vi "Circular Buffer(2D Wfm).vi"(7 "Buffer Size":T3, 8 "error in (no error)":errorcluster, 9 "Read Size":i32, 10 "Operation":T1, 11 "Data In":waveform(dbl)[](array[waveform])) -> (0 "error out":errorcluster, 1 "Elements Remaining":i32, 2 "Buffer Status":T2, 3 "Data Out":waveform(dbl)[](array[waveform]))   [LabVIEW 2016, in "Circular Buffer.lvlib"]
doc: "This VI implements a circular buffer which data can be written to and read from. There can only be one buffer per data type at once, but you can have multiple buffers of different types at the same time. For example, you can have a buffer of Wfm data types as well as I32s in the same VI. You cannot have two independent buffers of I32s."
uses:
  Circular Buffer.lvlib
  Controls/Circular Buffer Status.ctl
  Controls/Circular Buffer Operations.ctl
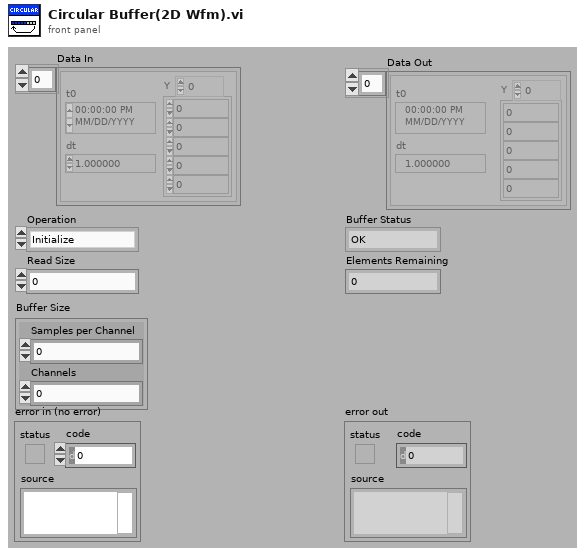
[diagram p1: front panel]
types:
  T1 = typedef "Circular Buffer.lvlib/Circular Buffer Operations.ctl" = enum16{"Initialize", "Get Backlog", "Write", "Read (continuous)", "Read (most recent)"}
  T2 = typedef "Circular Buffer.lvlib/Circular Buffer Status.ctl" = enum16{"OK", "Overflow", "Underflow"}
  T3 = cluster{"Samples per Channel":u32, "Channels":u32}
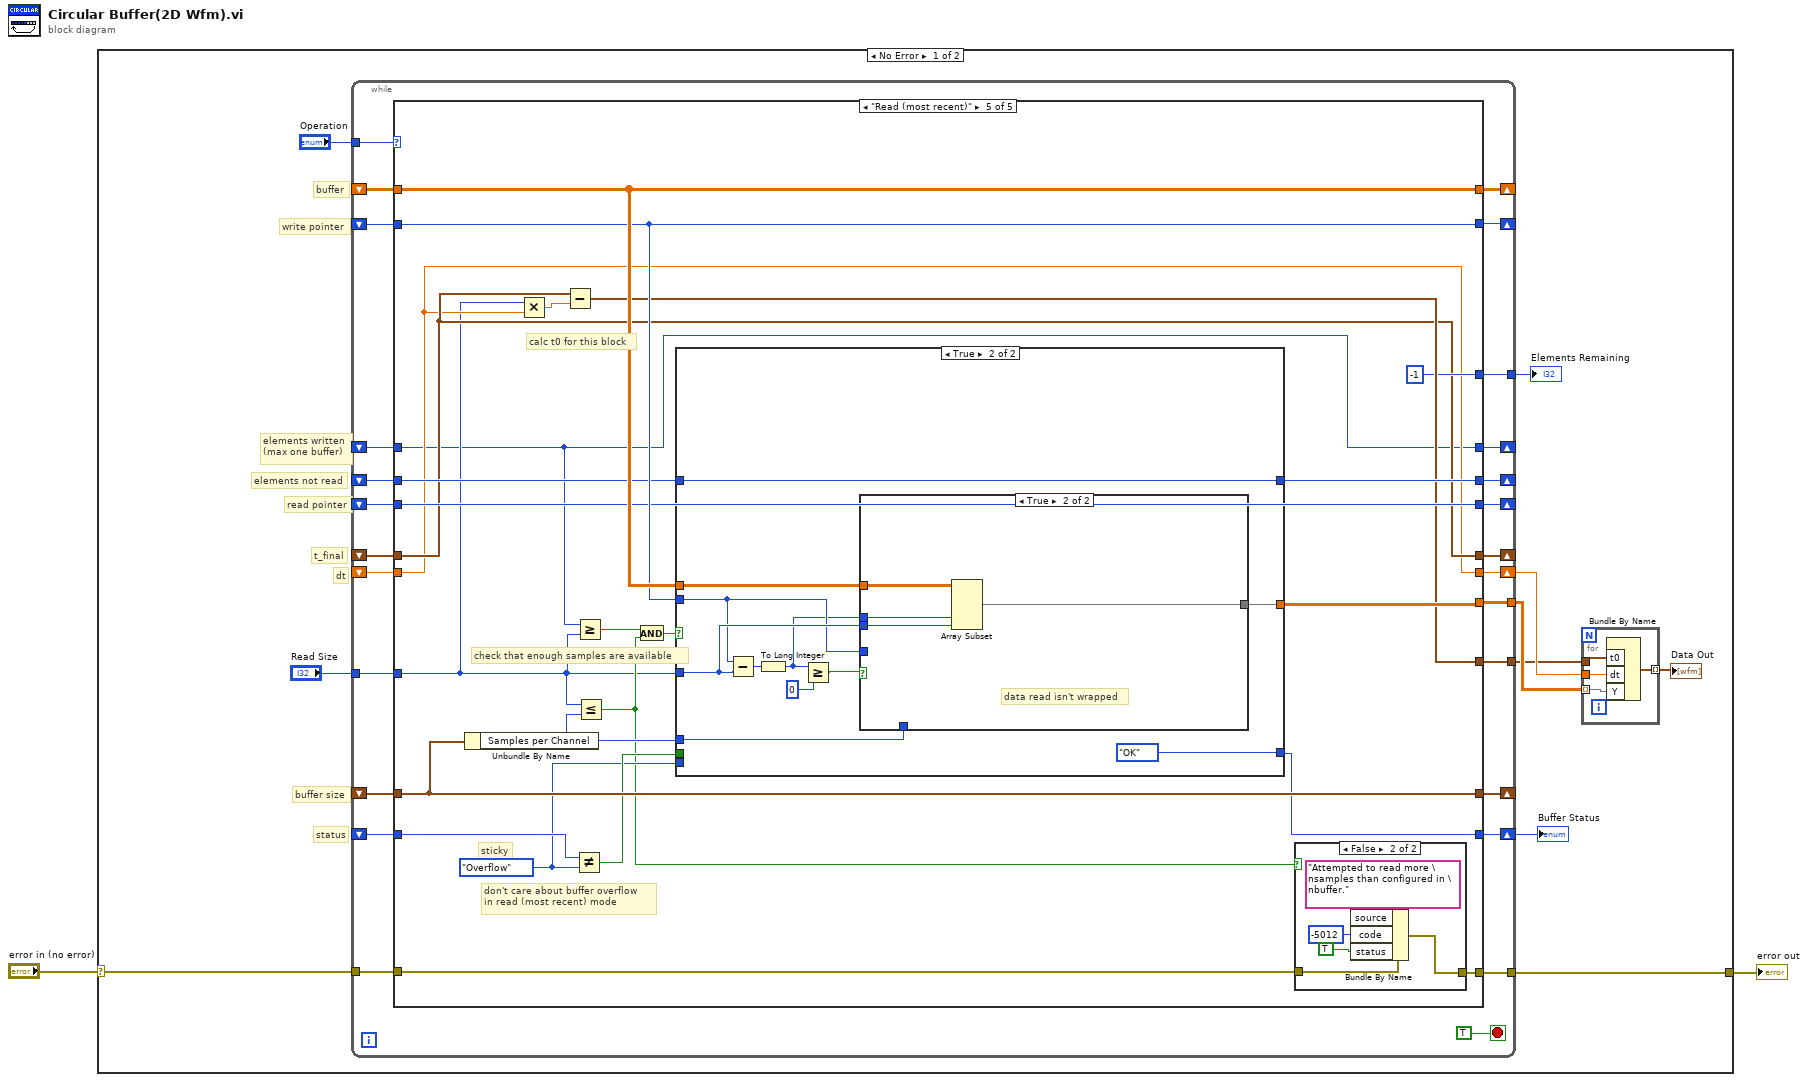
[diagram p0: block diagram]
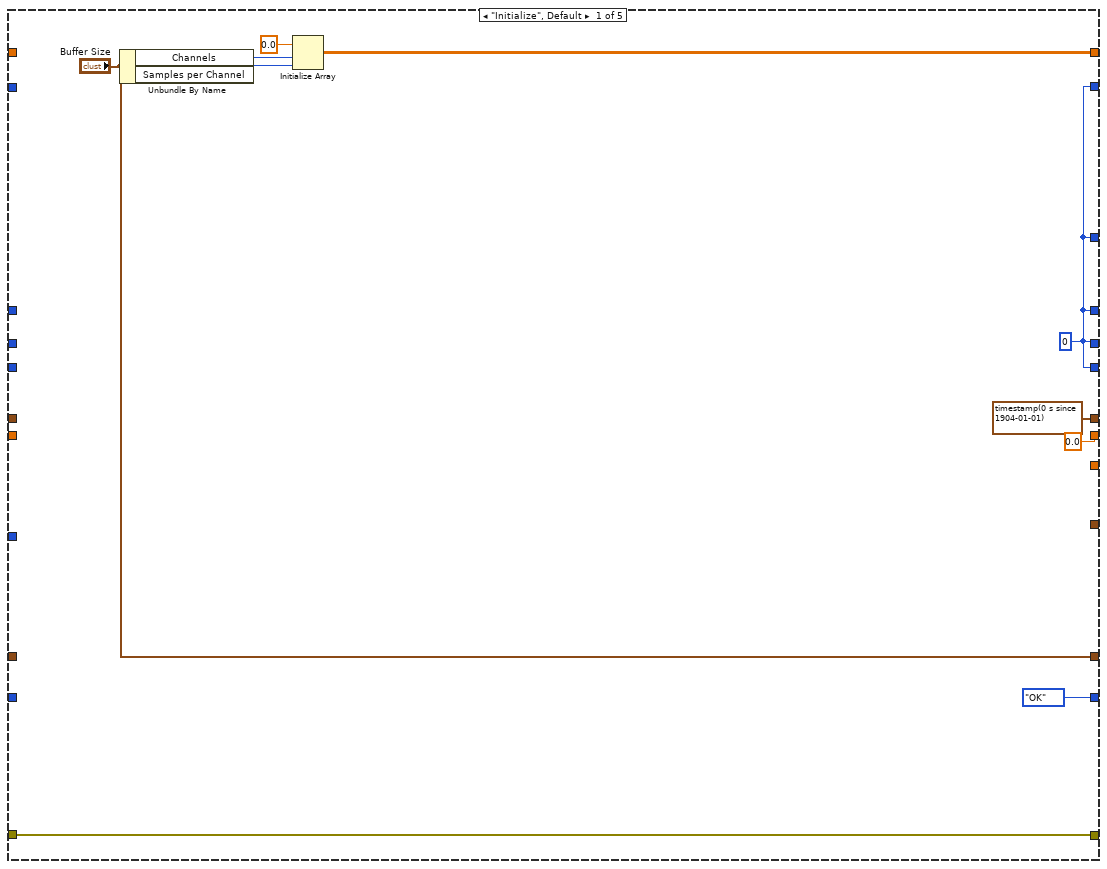
[diagram p2: hidden frame]
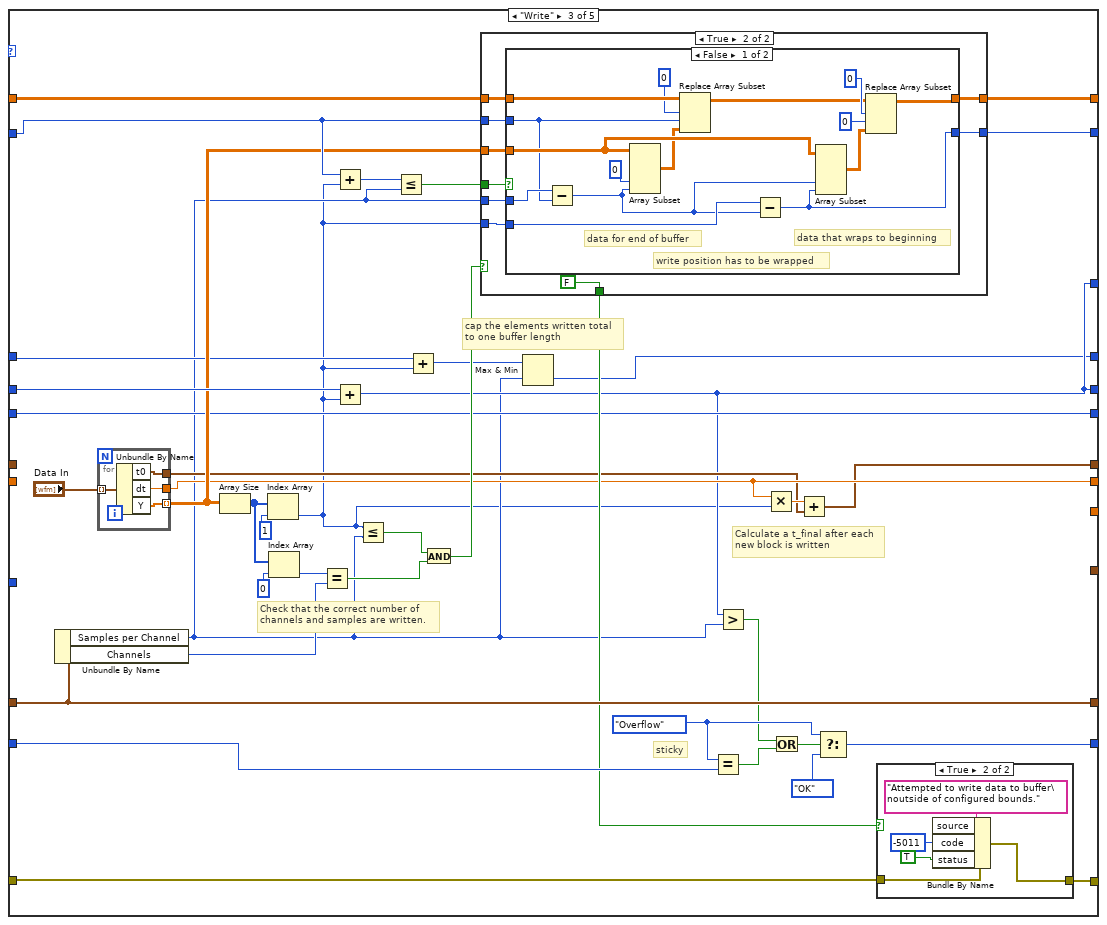
[diagram p4: hidden frame]
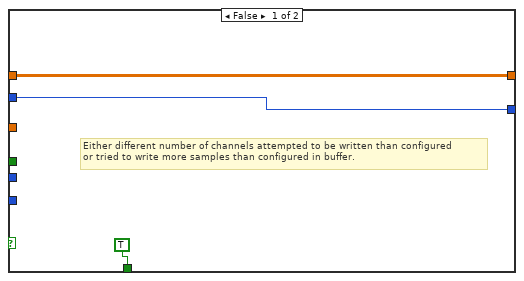
[diagram p6: hidden frame]
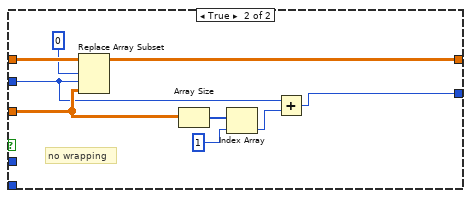
[diagram p7: hidden frame]
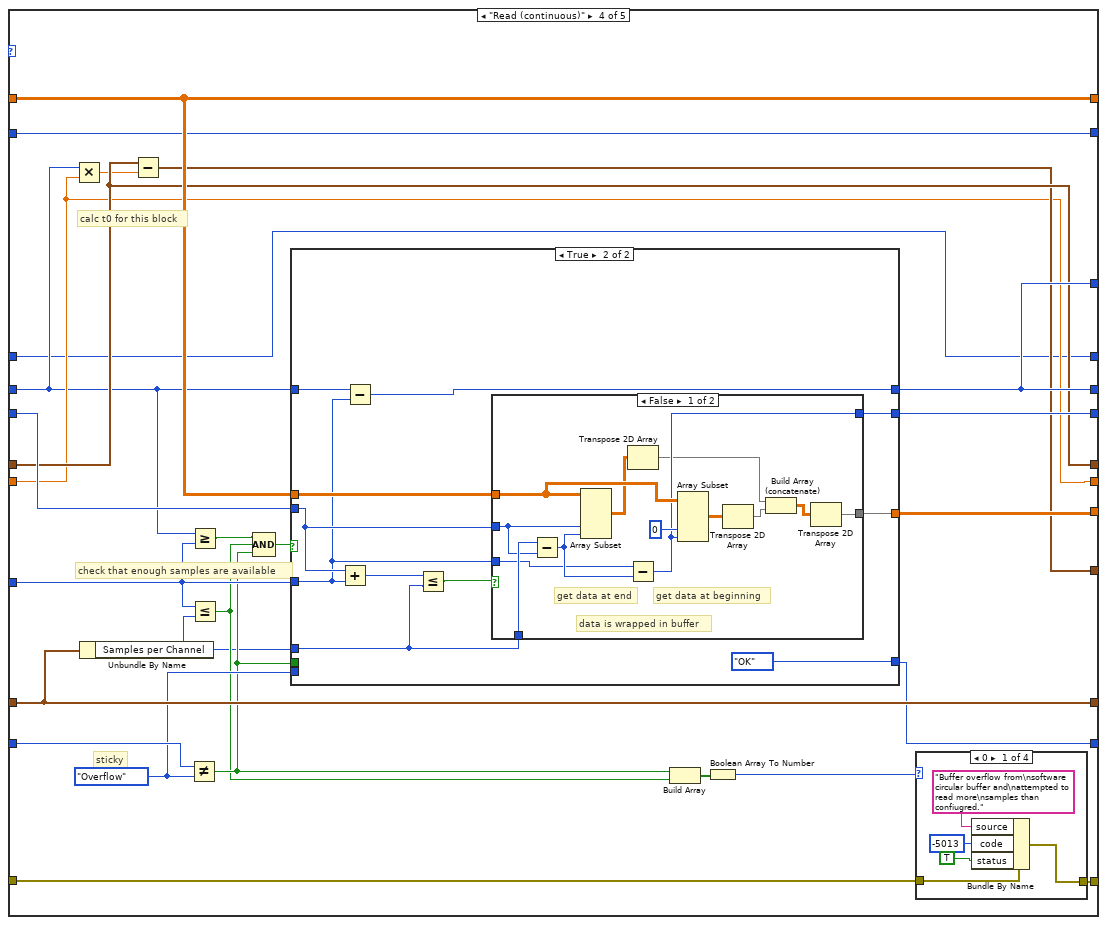
[diagram p8: hidden frame]
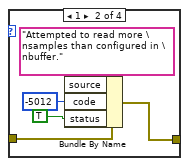
[diagram p9: hidden frame]
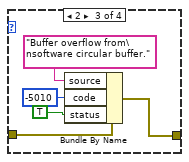
[diagram p10: hidden frame]
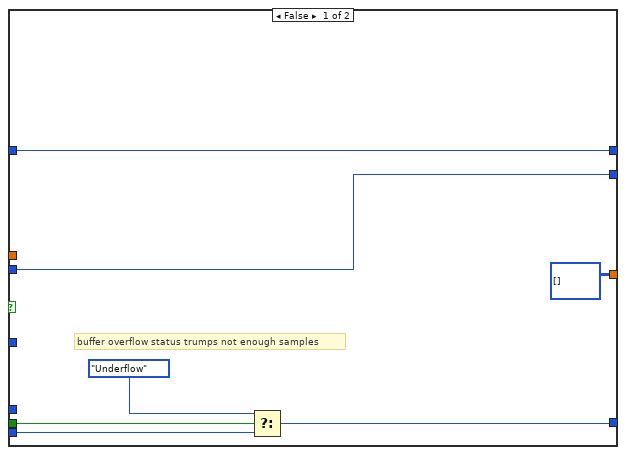
[diagram p12: hidden frame]
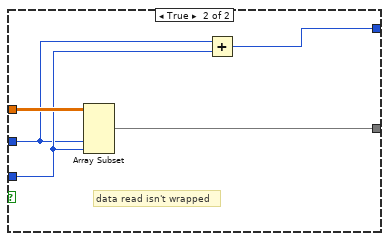
[diagram p13: hidden frame]
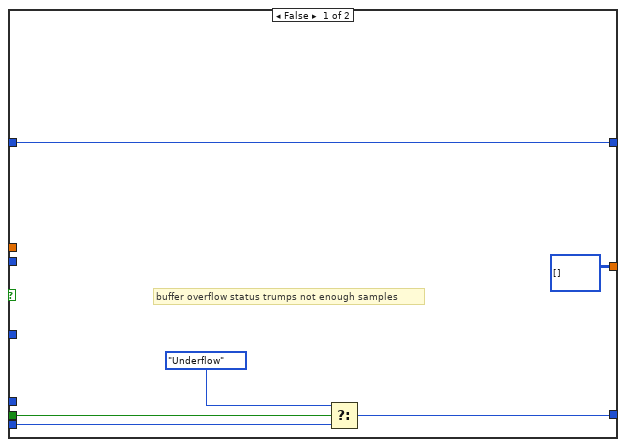
[diagram p15: hidden frame]
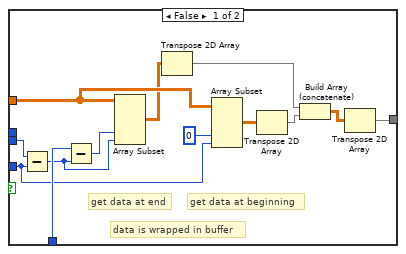
[diagram p16: hidden frame]
diagram:
  n1 = case shown="No Error" "error in (no error)" {
    selector: "error in (no error)" -> [w9 w290]
    tunnel: [w8 w290] -> w1
    frame No Error {
      # "elements written\n(max one buffer)"
      # "dt"
      # "t_final"
      # "write pointer"
      # "status"
      # "buffer size"
      # "read pointer"
      # "elements not read"
      # "buffer"
      n2 = while {
        tunnel: "Operation" -> [w41]
        shift-right: [w40] -> _
        shift-left: _ -> [w37]
        shift-right: [w39] -> _
        shift-left: _ -> [w36]
        shift-right: [w38] -> _
        shift-left: _ -> [w33]
        shift-right: [w35] -> _
        shift-left: _ -> [w34]
        tunnel: "Read Size" -> [w32]
        shift-right: [w31] -> w11
        shift-left: _ -> [w30]
        tunnel: [w29] -> w6
        tunnel: [w28] -> w8
        tunnel: w9 -> [w27]
        shift-right: [w26] -> _
        shift-left: _ -> [w25]
        shift-right: [w24] -> _
        shift-left: _ -> [w22]
        shift-right: [w23] -> w5
        shift-left: _ -> [w21]
        tunnel: [w20] -> w4
        tunnel: [w19] -> w3
        shift-right: [w18] -> _
        shift-left: _ -> [w17]
        stop <- TRUE stop-if-true
        n3 = case shown="\"Read (most recent)\"" w41 {
          tunnel: [w51 w61 w78 w173 w249] -> w40
          tunnel: [w43 w54 w68 w154 w244] -> w39
          tunnel: [w43 w56 w73 w156 w240] -> w38
          tunnel: w37 -> [_ w61 w77 w173 w249]
          tunnel: w36 -> [_ w54 w92 w149 w231]
          tunnel: ["Buffer Size" w55 w101 w172 w248] -> w35
          tunnel: w34 -> [_ w55 w101 w172 w248]
          tunnel: w33 -> [_ w56 w73 w169 w240]
          tunnel: w32 -> [_ _ _ w164 w228]
          tunnel: [Circular_Buffer_Status."OK" ("status") w60 w100 w168 w243] -> w31
          tunnel: w30 -> [_ w60 w97 w171 w247]
          tunnel: [_ _ _ w165 w242] -> w29
          tunnel: [w46 w62 w86 w167 w238] -> w28
          tunnel: w27 -> [w46 w62 w85 w166 w239]
          tunnel: [w43 w57 w74 w157 w241] -> w26
          tunnel: w25 -> [_ w57 w89 w157 w241]
          tunnel: [timestamp(0 s since 1904-01-01) ("t0") w59 w69 w153 w230] -> w24
          tunnel: [0.0 ("dt") w58 w71 w150 w229] -> w23
          tunnel: w22 -> [_ w59 _ w153 w230]
          tunnel: w21 -> [_ w58 _ w150 w229]
          tunnel: [_ _ _ w152 w233] -> w20
          tunnel: [w43 w54 w68 w154 -1] -> w19
          tunnel: [w43 w53 w64 w148 w226] -> w18
          tunnel: w17 -> [_ w53 w67 w148 w226]
          frame "Initialize", Default {
            w43 = 0 ("dimension size 2")
            n4 = Unbundle By Name("Buffer Size") -> ("Channels"=w48:u32, "Samples per Channel"=w47:u32)
            n5 = Initialize Array(0.0 ("element"), w48, w47) -> (w51:dbl[][])
          }
          frame "Get Backlog" {
          }
          frame "Write" {
            w96 = Circular_Buffer_Status."Overflow" ("status")
            # "cap the elements written total\nto one buffer length"
            # "Calculate a t_final after each\nnew block is written"
            # "Check that the correct number of\nchannels and samples are written."
            # "sticky"
            n6 = Unbundle By Name(w101) -> ("Samples per Channel"=w65:u32, "Channels"=w82:u32)
            n7 = for {
              tunnel: "Data In" -> [w105] mode=indexing
              tunnel: [w104] -> w75 mode=indexing
              tunnel: [w103] -> w71
              tunnel: [w102] -> w70
              n8 = Unbundle By Name(w105) -> ("t0"=w102:timestamp, "dt"=w103:dbl, "Y"=w104:dbl[])
            }
            n9 = Array Size(array=w75) -> (size(s)=w88:i32[])
            n10 = Index Array(array=w88, index=1) -> (element=w63:i32)
            n11 = Index Array(array=w88, index=0) -> (element=w83:i32)
            n12 = Equal?(x=w83, y=w82) -> (x = y?=w80:bool)
            n13 = Add(x=w89, y=w63) -> (x+y=w91:u32)
            n14 = Add(x=w92, y=w63) -> (x+y=w68:i32)
            n15 = Less Or Equal?(x=w63, y=w65) -> (x <= y?=w81:bool)
            n16 = Less Or Equal?(x=w91, y=w65) -> (x <= y?=w90:bool)
            n17 = Add(x=w67, y=w63) -> (x+y=w66:u32)
            n18 = And(x=w81, y=w80) -> (x .and. y?=w79:bool)
            n19 = case shown="True" w79 {
              tunnel: [w114 w123] -> w78
              tunnel: w90 -> [_ w122]
              tunnel: [w113 w121] -> w74
              tunnel: w89 -> [w113 w120]
              tunnel: w77 -> [w114 w119]
              tunnel: w75 -> [_ w118]
              tunnel: w63 -> [_ w117]
              tunnel: w65 -> [_ w116]
              tunnel: [TRUE FALSE] -> w84
              frame False {
                # "Either different number of channels attempted to be written than configured\nor tried to write more samples than configured in buffer."
              }
              frame True {
                n20 = case shown="False" w122 {
                  tunnel: w119 -> [w138 w147]
                  tunnel: [w133 w145] -> w123
                  tunnel: w120 -> [w127 w140]
                  tunnel: w118 -> [w131 w142]
                  tunnel: w116 -> [w128 _]
                  tunnel: w117 -> [w130 _]
                  tunnel: [w129 w139] -> w121
                  frame False {
                    # "data that wraps to beginning"
                    # "data for end of buffer"
                    # "write position has to be wrapped"
                    n21 = Subtract(x=w128, y=w127) -> (x-y=w126:u32)
                    n22 = Array Subset(array=w131, index (col)=0 ("index"), length (col)=w126) -> (w125:dbl[][])  [unwired: 2 in]
                    n23 = Replace Array Subset(array=w138, new element=w125, index (row)=0, index (col)=w127) -> (w134:dbl[][])
                    n24 = Subtract(x=w130, y=w126) -> (x-y=w129:u32)
                    n25 = Array Subset(array=w131, index (col)=w126, length (col)=w129) -> (w136:dbl[][])  [unwired: 2 in]
                    n26 = Replace Array Subset(array=w134, new element=w136, index (row)=0, index (col)=0 ("disabled index (col)")) -> (w133:dbl[][])
                  }
                  frame True {
                    # "no wrapping"
                    n27 = Replace Array Subset(array=w147, new element=w142, index (row)=0 ("disabled index (col)"), index (col)=w140) -> (w145:dbl[][])
                    n28 = Array Size(array=w142) -> (size(s)=w144:i32[])
                    n29 = Index Array(array=w144, index=1) -> (element=w141:i32)
                    n30 = Add(x=w140, y=w141) -> (x+y=w139:u32)
                  }
                }
              }
            }
            n31 = Max & Min(x=w66, y=w65) -> (min(x,y)=w64:u32)  [unwired: 1 out]
            n32 = Equal?(x=w96, y=w97) -> (x = y?=w99:bool)
            n33 = Greater?(x=w68, y=w65) -> (0:w94:bool)
            n34 = Multiply(x=w71, y=w63) -> (x*y=w72:dbl)
            n35 = Or(x=w94, y=w99) -> (x .or. y?=w98:bool)
            n36 = Add(x=w72, y=w70) -> (x+y=w69:timestamp)
            n37 = Select(t=w96, s=w98, f=Circular_Buffer_Status."OK" ("status")) -> (s? t:f=w100:T2)
            n38 = case shown="True" w84 {
              tunnel: w85 -> [w106 w111]
              tunnel: [w106 w110] -> w86
              frame False {
              }
              frame True {
                n39 = Bundle By Name(cluster=w111, "source"="Attempted to write data to buffer\noutside of configured bounds.", "code"=-5011, "status"=TRUE) -> (w110:errorcluster)
              }
            }
          }
          frame "Read (continuous)" {
            w170 = Circular_Buffer_Status."Overflow" ("status")
            # "calc t0 for this block"
            # "check that enough samples are available"
            # "sticky"
            n40 = Multiply(x=w149, y=w150) -> (x*y=w151:dbl)
            n41 = Unbundle By Name(w172) -> ("Samples per Channel"=w155:u32)
            n42 = Subtract(x=w153, y=w151) -> (x-y=w152:timestamp)
            n43 = Not Equal?(x=w171, y=w170) -> (x != y?=w161:bool)
            n44 = Greater Or Equal?(x=w149, y=w164) -> (x >= y?=w163:bool)
            n45 = Less Or Equal?(x=w164, y=w155) -> (x <= y?=w160:bool)
            n46 = Compound Arithmetic op=AND(w163, w160, w161) -> (w162:bool)
            n47 = case shown="True" w162 {
              tunnel: w169 -> [w191 w200]
              tunnel: w173 -> [_ w206]
              tunnel: w164 -> [_ w198]
              tunnel: w155 -> [_ w201]
              tunnel: [w195 Circular_Buffer_Status."OK" ("status")] -> w168
              tunnel: w161 -> [w196 _]
              tunnel: w170 -> [w194 _]
              tunnel: w149 -> [w192 w199]
              tunnel: [w192 w197] -> w154
              tunnel: [w191 w202] -> w156
              tunnel: [i32[][] [] w203] -> w165
              frame False {
                # "buffer overflow status trumps not enough samples"
                n48 = Select(t=Circular_Buffer_Status."Underflow" ("status"), s=w196, f=w194) -> (s? t:f=w195:T2)
              }
              frame True {
                n49 = Add(x=w200, y=w198) -> (x+y=w205:u32)
                n50 = Subtract(x=w199, y=w198) -> (x-y=w197:i32)
                n51 = Less Or Equal?(x=w205, y=w201) -> (x <= y?=w204:bool)
                n52 = case shown="False" w204 {
                  tunnel: w206 -> [w219 w225]
                  tunnel: w200 -> [w215 w222]
                  tunnel: w198 -> [w208 w223]
                  tunnel: [w210 w224] -> w203
                  tunnel: [w216 w221] -> w202
                  tunnel: w201 -> [w220 _]
                  frame False {
                    # "get data at beginning"
                    # "get data at end"
                    # "data is wrapped in buffer"
                    n53 = Subtract(x=w220, y=w215) -> (x-y=w217:u32)
                    n54 = Array Subset(array=w219, index (col)=w215, length (col)=w217) -> (w214:dbl[][])  [unwired: 2 in]
                    n55 = Transpose 2D Array(2D array=w214) -> (transposed array=w212:dbl[][])
                    n56 = Subtract(x=w208, y=w217) -> (x-y=w216:u32)
                    n57 = Array Subset(array=w219, index (col)=0 ("index"), length (col)=w216) -> (w213:dbl[][])  [unwired: 2 in]
                    n58 = Transpose 2D Array(2D array=w213) -> (transposed array=w211:dbl[][])
                    n59 = Build Array (concatenate)(w212, w211) -> (w209:dbl[][])
                    n60 = Transpose 2D Array(2D array=w209) -> (transposed array=w210:dbl[][])
                  }
                  frame True {
                    # "data read isn't wrapped"
                    n61 = Array Subset(array=w225, index (col)=w222, length (col)=w223) -> (w224:dbl[][])  [unwired: 2 in]
                    n62 = Add(x=w222, y=w223) -> (x+y=w221:u32)
                  }
                }
              }
            }
            n63 = Build Array(w161, w160) -> (w159:bool[])
            n64 = Boolean Array To Number(Boolean array=w159) -> (number=w158:u32)
            n65 = case shown="0" w158 {
              tunnel: w166 -> [w178 w183 w188 w189]
              tunnel: [w177 w182 w187 w189] -> w167
              frame 0 {
                n66 = Bundle By Name(cluster=w178, "source"="Buffer overflow from\nsoftware circular buffer and\nattempted to read more\nsamples than confiugred.", "code"=-5013, "status"=TRUE) -> (w177:errorcluster)
              }
              frame 1 {
                n67 = Bundle By Name(cluster=w183, "source"="Attempted to read more \nsamples than configured in \nbuffer.", "code"=-5012, "status"=TRUE) -> (w182:errorcluster)
              }
              frame 2 {
                n68 = Bundle By Name(cluster=w188, "source"="Buffer overflow from\nsoftware circular buffer.", "code"=-5010, "status"=TRUE) -> (w187:errorcluster)
              }
              frame 3, Default {
              }
            }
          }
          frame "Read (most recent)" {
            w245 = Circular_Buffer_Status."Overflow" ("status")
            # "calc t0 for this block"
            # "don't care about buffer overflow\nin read (most recent) mode"
            # "check that enough samples are available"
            # "sticky"
            n69 = Unbundle By Name(w248) -> ("Samples per Channel"=w237:u32)
            n70 = Multiply(x=w228, y=w229) -> (x*y=w227:dbl)
            n71 = Subtract(x=w230, y=w227) -> (x-y=w233:timestamp)
            n72 = Not Equal?(x=w247, y=w245) -> (x != y?=w246:bool)
            n73 = Greater Or Equal?(x=w226, y=w228) -> (x >= y?=w235:bool)
            n74 = Less Or Equal?(x=w228, y=w237) -> (x <= y?=w234:bool)
            n75 = And(x=w235, y=w234) -> (x .and. y?=w236:bool)
            n76 = case shown="True" w236 {
              tunnel: w241 -> [_ w264]
              tunnel: w249 -> [_ w270]
              tunnel: w228 -> [_ w266]
              tunnel: w237 -> [_ w267]
              tunnel: [w260 Circular_Buffer_Status."OK" ("status")] -> w243
              tunnel: w246 -> [w261 _]
              tunnel: w245 -> [w259 _]
              tunnel: w231 -> [w257 w271]
              tunnel: [w257 w271] -> w244
              tunnel: [i32[][] [] w268] -> w242
              frame False {
                # "buffer overflow status trumps not enough samples"
                n77 = Select(t=Circular_Buffer_Status."Underflow" ("status"), s=w261, f=w259) -> (s? t:f=w260:T2)
              }
              frame True {
                n78 = Subtract(x=w264, y=w266) -> (x-y=w263:u32)
                n79 = To Long Integer(number=w263) -> (32bit integer=w262:i32)
                n80 = Greater Or Equal?(x=w262, y=0) -> (x >= y?=w269:bool)
                n81 = case shown="True" w269 {
                  tunnel: w270 -> [w284 w289]
                  tunnel: [w278 w288] -> w268
                  tunnel: w267 -> [w285 _]
                  tunnel: w262 -> [_ w287]
                  tunnel: w266 -> [w276 w286]
                  tunnel: w264 -> [w273 _]
                  frame False {
                    # "get data at beginning"
                    # "get data at end"
                    # "data is wrapped in buffer"
                    n82 = Subtract(x=w276, y=w273) -> (x-y=w274:u32)
                    n83 = Subtract(x=w285, y=w274) -> (x-y=w275:u32)
                    n84 = Array Subset(array=w284, index (col)=w275, length (col)=w274) -> (w282:dbl[][])  [unwired: 2 in]
                    n85 = Transpose 2D Array(2D array=w282) -> (transposed array=w280:dbl[][])
                    n86 = Array Subset(array=w284, index (col)=0 ("index"), length (col)=w273) -> (w281:dbl[][])  [unwired: 2 in]
                    n87 = Transpose 2D Array(2D array=w281) -> (transposed array=w279:dbl[][])
                    n88 = Build Array (concatenate)(w280, w279) -> (w277:dbl[][])
                    n89 = Transpose 2D Array(2D array=w277) -> (transposed array=w278:dbl[][])
                  }
                  frame True {
                    # "data read isn't wrapped"
                    n90 = Array Subset(array=w289, index (col)=w287, length (col)=w286) -> (w288:dbl[][])  [unwired: 2 in]
                  }
                }
              }
            }
            n91 = case shown="False" w234 {
              tunnel: w239 -> [w250 w255]
              tunnel: [w250 w254] -> w238
              frame True {
              }
              frame False {
                n92 = Bundle By Name(cluster=w255, "source"="Attempted to read more \nsamples than configured in \nbuffer.", "code"=-5012, "status"=TRUE) -> (w254:errorcluster)
              }
            }
          }
        }
      }
      "Elements Remaining" <- w3
      "Buffer Status" <- w11
      n93 = for {
        tunnel: [w16] -> w7 mode=indexing
        tunnel: w6 -> [w15] mode=indexing
        tunnel: w5 -> [w14]
        tunnel: w4 -> [w13]
        n94 = Bundle By Name("t0"=w13, "dt"=w14, "Y"=w15) -> (w16:waveform(dbl))  [unwired: 1 out]
      }
      "Data Out" <- w7
    }
    frame Error {
    }
  }
  "error out" <- w1
